vi "PCO_Description_Intensified.vi"() -> (0 "PCO_Description_Intensified":T1 {"dwFlagsIntensifiedDESC" format="%x"}, 1 "PCO_Description_Intensified_Raw":T2, 2 "Length":u16, 3 "Raw_Length":u16)   [LabVIEW 2019, in "SDK.lvlib" / "Structures.lvlib"]
doc: "Use this template to build a VI to use as a subVI."
uses:
  Structures.lvlib
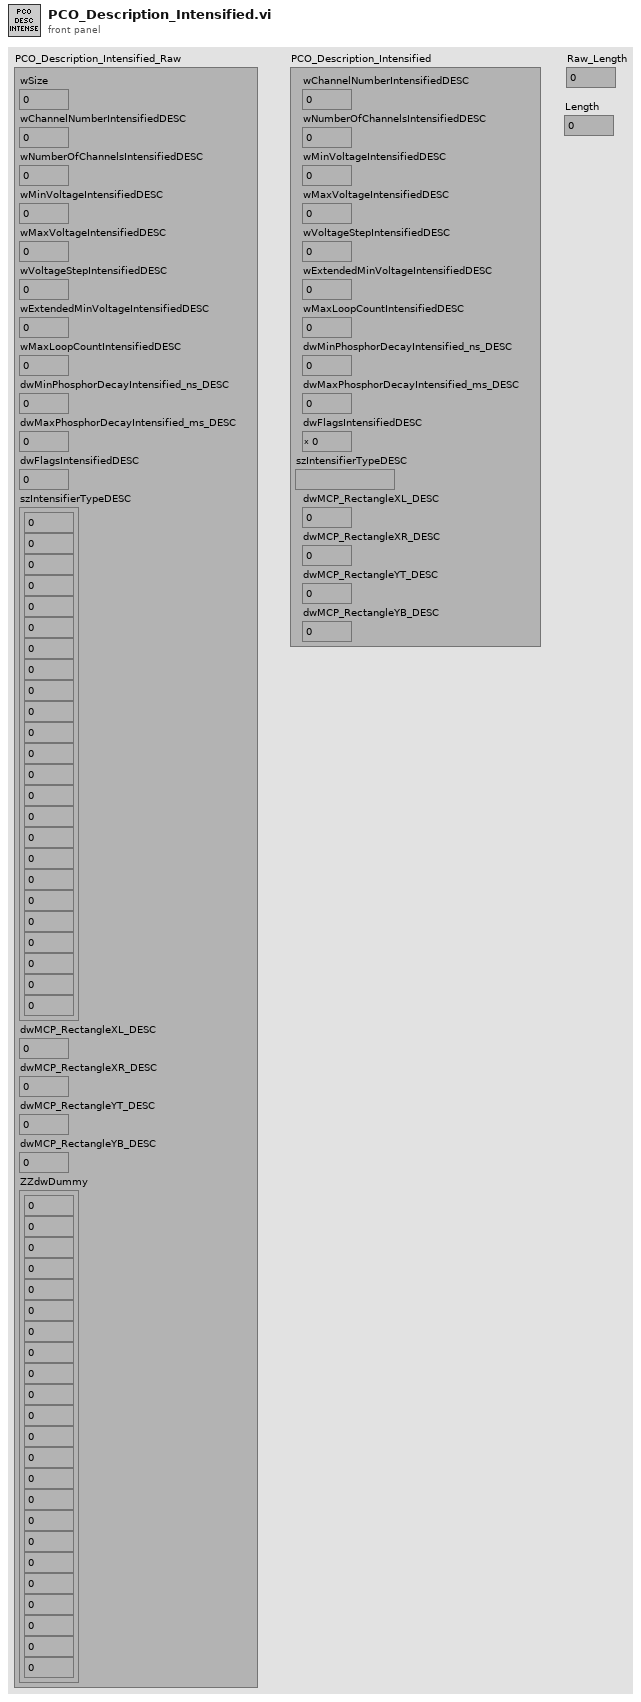
[diagram p1: front panel]
types:
  T1 = cluster{"wChannelNumberIntensifiedDESC":u16, "wNumberOfChannelsIntensifiedDESC":u16, "wMinVoltageIntensifiedDESC":u16, "wMaxVoltageIntensifiedDESC":u16, "wVoltageStepIntensifiedDESC":u16, "wExtendedMinVoltageIntensifiedDESC":u16, "wMaxLoopCountIntensifiedDESC":u16, "dwMinPhosphorDecayIntensified_ns_DESC":u32, "dwMaxPhosphorDecayIntensified_ms_DESC":u32, "dwFlagsIntensifiedDESC":u32, "szIntensifierTypeDESC":string, "dwMCP_RectangleXL_DESC":u32, "dwMCP_RectangleXR_DESC":u32, "dwMCP_RectangleYT_DESC":u32, "dwMCP_RectangleYB_DESC":u32}
  T2 = cluster{"wSize":u16, "wChannelNumberIntensifiedDESC":u16, "wNumberOfChannelsIntensifiedDESC":u16, "wMinVoltageIntensifiedDESC":u16, "wMaxVoltageIntensifiedDESC":u16, "wVoltageStepIntensifiedDESC":u16, "wExtendedMinVoltageIntensifiedDESC":u16, "wMaxLoopCountIntensifiedDESC":u16, "dwMinPhosphorDecayIntensified_ns_DESC":u32, "dwMaxPhosphorDecayIntensified_ms_DESC":u32, "dwFlagsIntensifiedDESC":u32, "szIntensifierTypeDESC":cluster{u8, u8, u8, u8, u8, u8, u8, u8, u8, u8, u8, u8, u8, u8, u8, u8, u8, u8, u8, u8, u8, u8, u8, u8}, "dwMCP_RectangleXL_DESC":u32, "dwMCP_RectangleXR_DESC":u32, "dwMCP_RectangleYT_DESC":u32, "dwMCP_RectangleYB_DESC":u32, "ZZdwDummy":cluster{u32, u32, u32, u32, u32, u32, u32, u32, u32, u32, u32, u32, u32, u32, u32, u32, u32, u32, u32, u32, u32, u32, u32}}
  T3 = cluster{u8, u8, u8, u8, u8, u8, u8, u8, u8, u8, u8, u8, u8, u8, u8, u8, u8, u8, u8, u8, u8, u8, u8, u8}
  T4 = cluster{u32, u32, u32, u32, u32, u32, u32, u32, u32, u32, u32, u32, u32, u32, u32, u32, u32, u32, u32, u32, u32, u32, u32}
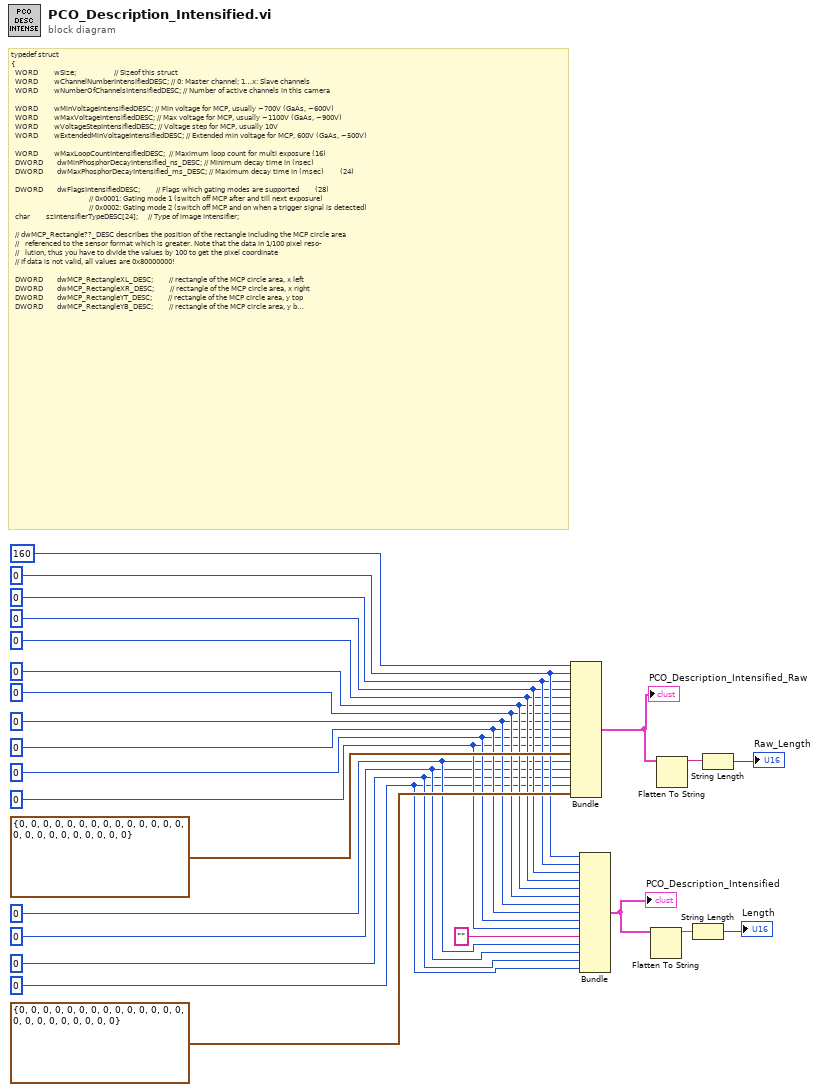
[diagram p0: block diagram]
diagram:
  w1 = u32 0 ("dwMCP_RectangleYB_DESC")
  w2 = u32 0 ("dwMCP_RectangleYT_DESC")
  w3 = u32 0 ("dwMCP_RectangleXR_DESC")
  w4 = u32 0 ("dwMCP_RectangleXL_DESC")
  w6 = u32 0 ("dwFlagsIntensifiedDESC")
  w7 = u32 0 ("dwMaxPhosphorDecayIntensified_ms_DESC")
  w8 = u32 0 ("dwMinPhosphorDecayIntensified_ns_DESC")
  w9 = u16 0 ("wMaxLoopCountIntensifiedDESC")
  w10 = u16 0 ("wExtendedMinVoltageIntensifiedDESC")
  w11 = u16 0 ("wVoltageStepIntensifiedDESC")
  w12 = u16 0 ("wMaxVoltageIntensifiedDESC")
  w13 = u16 0 ("wMinVoltageIntensifiedDESC")
  w14 = u16 0 ("wNumberOfChannelsIntensifiedDESC")
  w15 = u16 0 ("wChannelNumberIntensifiedDESC")
  # "typedef struct\n{\n  WORD        wSize;                   // Sizeof this struct\n  WORD        wChannelNumberIntensifiedDESC; // 0: Master channel; 1…x: Slave channels\n  WORD        wNumberOfChannelsIntensifiedDESC; // Number of active channels in this camera\n\n  WORD        wMinVoltageIntensifiedDESC; // Min voltage for MCP, usually ~700V (GaAs, ~600V)\n  WORD        wMaxVoltageIntensifiedDESC; // Max voltage for MCP, usually ~1100V (GaAs, ~900V)\n  WORD        wVoltageStepIntensifiedDESC; // Voltage step for MCP, usually 10V\n  WORD        wExtendedMinVoltageIntensifiedDESC; // Extended min voltage for MCP, 600V (GaAs, ~500V)\n\n  WORD        wMaxLoopCountIntensifiedDESC;  // Maximum loop count for multi exposure (16)\n  DWORD       dwMinPhosphorDecayIntensified_ns_DESC; // Minimum decay time in (nsec)\n  DWORD       dwMaxPhosphorDecayIntensified_ms_DESC; // Maximum decay time in (msec)        (24)\n\n  DWORD       dwFlagsIntensifiedDESC;        // Flags which gating modes are supported        (28)\n                                       // 0x0001: Gating mode 1 (switch off MCP after and till next exposure)\n                                       // 0x0002: Gating mode 2 (switch off MCP and on when a trigger signal is detected)\n  char        szIntensifierTypeDESC[24];     // Type of image intensifier;\n\n  // dwMCP_Rectangle??_DESC describes the position of the rectangle including the MCP circle area \n  //   referenced to the sensor format which is greater. Note that the data in 1/100 pixel reso-\n  //   lution, thus you have to divide the values by 100 to get the pixel coordinate\n  // If data is not valid, all values are 0x80000000!\n\n  DWORD       dwMCP_RectangleXL_DESC;        // rectangle of the MCP circle area, x left\n  DWORD       dwMCP_RectangleXR_DESC;        // rectangle of the MCP circle area, x right \n  DWORD       dwMCP_RectangleYT_DESC;        // rectangle of the MCP circle area, y top\n  DWORD       dwMCP_RectangleYB_DESC;        // rectangle of the MCP circle area, y bottom (68)\n\n  DWORD       ZZdwDummy[23];                                                          //(160)\n} PCO_Description_Intensified;"
  n1 = Bundle("wSize"=u16 160, "wChannelNumberIntensifiedDESC"=w15, "wNumberOfChannelsIntensifiedDESC"=w14, "wMinVoltageIntensifiedDESC"=w13, "wMaxVoltageIntensifiedDESC"=w12, "wVoltageStepIntensifiedDESC"=w11, "wExtendedMinVoltageIntensifiedDESC"=w10, "wMaxLoopCountIntensifiedDESC"=w9, "dwMinPhosphorDecayIntensified_ns_DESC"=w8, "dwMaxPhosphorDecayIntensified_ms_DESC"=w7, "dwFlagsIntensifiedDESC"=w6, "szIntensifierTypeDESC"=T3 {0, 0, 0, 0, 0, 0, 0, 0, 0, 0, 0, 0, 0, 0, 0, 0, 0, 0, 0, 0, 0, 0, 0, 0}, "dwMCP_RectangleXL_DESC"=w4, "dwMCP_RectangleXR_DESC"=w3, "dwMCP_RectangleYT_DESC"=w2, "dwMCP_RectangleYB_DESC"=w1, "ZZdwDummy"=T4 {0, 0, 0, 0, 0, 0, 0, 0, 0, 0, 0, 0, 0, 0, 0, 0, 0, 0, 0, 0, 0, 0, 0}) -> (w19:T2)  [unwired: 1 in]
  "PCO_Description_Intensified_Raw" <- w19
  n2 = Bundle("wChannelNumberIntensifiedDESC"=w15, "wNumberOfChannelsIntensifiedDESC"=w14, "wMinVoltageIntensifiedDESC"=w13, "wMaxVoltageIntensifiedDESC"=w12, "wVoltageStepIntensifiedDESC"=w11, "wExtendedMinVoltageIntensifiedDESC"=w10, "wMaxLoopCountIntensifiedDESC"=w9, "dwMinPhosphorDecayIntensified_ns_DESC"=w8, "dwMaxPhosphorDecayIntensified_ms_DESC"=w7, "dwFlagsIntensifiedDESC"=w6, "szIntensifierTypeDESC"="", "dwMCP_RectangleXL_DESC"=w4, "dwMCP_RectangleXR_DESC"=w3, "dwMCP_RectangleYT_DESC"=w2, "dwMCP_RectangleYB_DESC"=w1) -> (w24:T1)  [unwired: 1 in]
  "PCO_Description_Intensified" <- w24
  n3 = Flatten To String(anything=w24) -> (data string=w23:string)  [unwired: 3 in, 2 out]
  n4 = Flatten To String(anything=w19) -> (data string=w22:string)  [unwired: 3 in, 2 out]
  n5 = String Length(string=w23) -> (length=→"Length":i32)
  n6 = String Length(string=w22) -> (length=→"Raw_Length":i32)
